vi "WaveformConcatenate.vi"(0 "Before":waveform(dbl)={"t0"=timestamp(287281825.734 s since 1904-01-01), "dt"=0.001, "Y"=array[1000 elements], "attributes"=variant("Name"=variant(string "FringeTracker[0].CompleteControllerSet.ControllerData.ChannelData[0].CalibratedBinData[0]"))}, 1 "After":waveform(dbl)={"t0"=timestamp(287281826.734 s since 1904-01-01), "dt"=0.001, "Y"=array[1000 elements], "attributes"=variant("Name"=variant(string "FringeTracker[0].CompleteControllerSet.ControllerData.ChannelData[0].CalibratedBinData[0]"))}) -> (2 "Before After":waveform(dbl))   [LabVIEW 2009]
uses:
  <vilib>/Waveform/WDTOps.llb/WDT Get Final Time Value DBL.vi
  <vilib>/Waveform/WDTOps.llb/WDT Waveform Duration DBL.vi
  <vilib>/Waveform/WDTOps.llb/WDT Append Waveforms DBL.vi
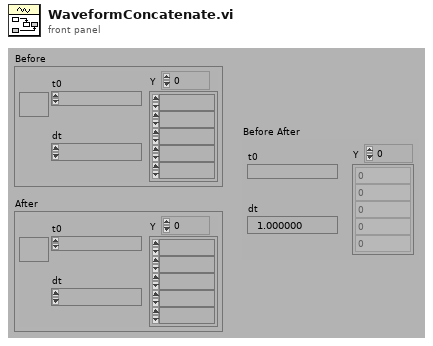
[diagram p1: front panel]
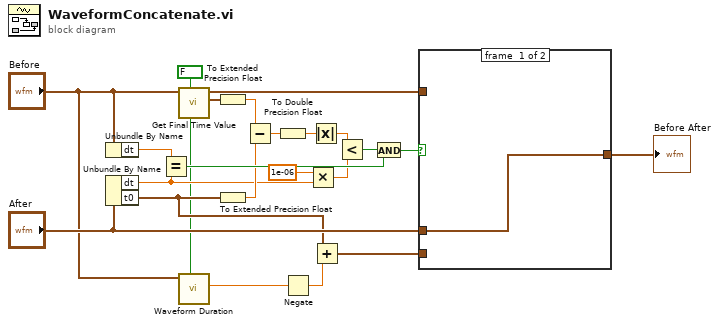
[diagram p0: block diagram]
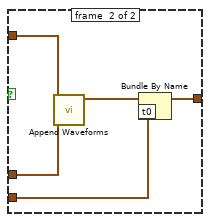
[diagram p2: hidden frame]
diagram:
  w2 = FALSE ("open interval? (T)")
  n1 = Unbundle By Name("Before") -> ("dt"=w22:dbl)
  n2 = Unbundle By Name("After") -> ("dt"=w11:dbl, "t0"=w6:timestamp)
  n3 = Equal?(x=w22, y=w11) -> (x = y?=w21:bool)
  n4 = call-poly <vilib>:"Get Final Time Value.vi"("open interval? (T)"=w2, "waveform in"="Before") -> ("tf"=w15:timestamp, "waveform out"=w20:waveform(dbl))  [unwired: 1 in, 7 out]
  n5 = call-poly <vilib>:"Waveform Duration.vi"("open interval? (T)"=w2, "waveform in"="Before") -> ("duration"=w5:dbl)  [unwired: 1 in, 8 out]
  n6 = To Extended Precision Float(1:w15) -> (0:w14:ext)
  n7 = To Extended Precision Float(1:w6) -> (0:w13:ext)
  n8 = Subtract(x=w14, y=w13) -> (x-y=w12:ext)
  n9 = To Double Precision Float(number=w12) -> (double precision float=w8:dbl)
  n10 = Negate(x=w5) -> (-x=w4:dbl)
  n11 = Multiply(x=1e-06, y=w11) -> (x*y=w9:dbl)
  n12 = Absolute Value(x=w8) -> (abs(x)=w1:dbl)
  n13 = Add(x=w6, y=w4) -> (x+y=w3:timestamp)
  n14 = Less?(x=w1, y=w9) -> (x < y?=w7:bool)
  n15 = And(x=w7, y=w21) -> (x .and. y?=w19:bool)
  n16 = case shown="True" w19 {
    tunnel: "After" -> [w23 w27]
    tunnel: w20 -> [_ w28]
    tunnel: [w23 w25] -> w16
    tunnel: w3 -> [_ w24]
    frame #0 {
    }
    frame #1 {
      n17 = call-poly <vilib>:"Append Waveforms.vi"("waveform B"=w27, "waveform A"=w28) -> ("waveform out"=w26:waveform(dbl))  [unwired: 1 in, 8 out]
      n18 = Bundle By Name(cluster=w26, "t0"=w24) -> (w25:waveform(dbl))
    }
  }
  "Before After" <- w16
